vi "KG set concentration mode.vi"(8 "Fehler (Eingang, kein Fehler)":errorcluster, 9 "mode":dbl, 10 "pump":u32, 11 "VISA-Ressourcenname":refnum<visa-resource-name>) -> (0 "Fehler (Ausgang)":errorcluster, 2 "Kommando gesendet":string, 3 "VISA-Ressourcenname (Ausgang)":refnum<visa-resource-name>)   [LabVIEW 2020, in "Linearisierung v2.lvlib" / "Gasteiler.lvlib" / "HovaCAL_Interface.lvlib" / "KGN.lvlib" / "set.lvlib"]
uses:
  set.lvlib
  KGN.lvlib
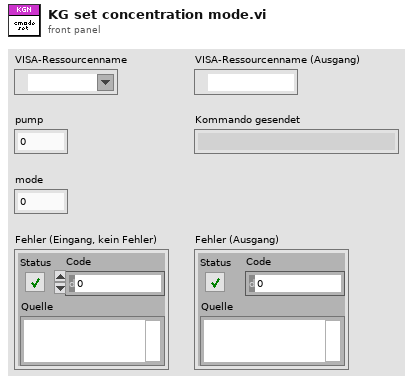
[diagram p1: front panel]
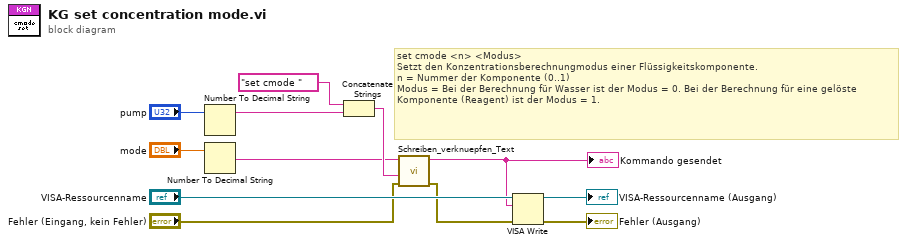
[diagram p0: block diagram]
diagram:
  # "set cmode <n> <Modus>\nSetzt den Konzentrationsberechnungmodus einer Flüssigkeitskomponente.\nn = Nummer der Komponente (0..1)\nModus = Bei der Berechnung für Wasser ist der Modus = 0. Bei der Berechnung für eine gelöste\nKomponente (Reagent) ist der Modus = 1."
  n1 = Number To Decimal String(number="pump") -> (decimal integer string=w7:string)  [unwired: 1 in]
  n2 = Number To Decimal String(number="mode") -> (decimal integer string=w1:string)  [unwired: 1 in]
  n3 = Concatenate Strings("set cmode " ("Schreibpuffer"), w7) -> (w4:string)
  n4 = call "Schreiben_verknuepfen_Text.vi"("error in (no error)"="Fehler (Eingang, kein Fehler)", "Order"=w4, "parameter"=w1) -> ("error out"=w5:errorcluster, "Verknüpfter String"=w3:string)  [unwired: 7 in]
  "Kommando gesendet" <- w3
  n5 = VISA Write(VISA resource name="VISA-Ressourcenname", write buffer=w3, error in (no error)=w5) -> (VISA resource name out=→"VISA-Ressourcenname (Ausgang)":refnum<visa-resource-name>, error out=→"Fehler (Ausgang)":errorcluster)  [unwired: 1 out]
